vi "Calculate Forces.vi"(7 "Integrator Reset":bool, 8 "error in (no error)":errorcluster, 10 "Vessel in":refnum<class "Vessel.lvclass">, 11 "Joystick Controller in":refnum<class "Joystick Controller.lvclass">) -> (0 "error out":errorcluster, 2 "Vessel out":refnum<class "Vessel.lvclass">, 3 "Joystick Controller out":refnum<class "Joystick Controller.lvclass">)   [LabVIEW 2014, in "Controller Library.lvlib" / "Joystick Controller.lvclass"]
doc: "This VI calculates the forces in each controlled degree of freedom direction to follow a desired path or point."
uses:
  Joystick Controller.lvclass
  ROV/Vessel.lvclass
  <vilib>/addons/control/pid/pid.llb/PID (DBL).vi
  Supervisor/Supervisor.lvclass
  <vilib>/addons/control/pid/NI_PID_pid.lvlib
panel:
  in  "PID gains depth":T1={"proportional gain (Kc)"=500.0, "integral time (Ti, min)"=0.83, "derivative time (Td, min)"=0.01} {"derivative time (Td, min)" format="%.3f"; "integral time (Ti, min)" format="%.3f"; "proportional gain (Kc)" format="%.3f"}
  in  "PID gains head":T1={"proportional gain (Kc)"=150.0, "integral time (Ti, min)"=0.5, "derivative time (Td, min)"=0.008} {"derivative time (Td, min)" format="%.3f"; "integral time (Ti, min)" format="%.3f"; "proportional gain (Kc)" format="%.3f"}
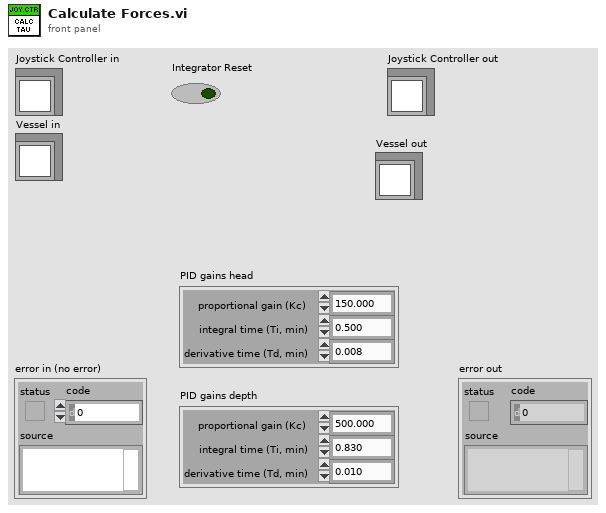
[diagram p1: front panel]
types:
  T1 = cluster{"proportional gain (Kc)":dbl, "integral time (Ti, min)":dbl, "derivative time (Td, min)":dbl}
  T2 = cluster{"Button 1":bool, "Button 2":bool, "Button 3":bool, "Button 4":bool, "Button 5":bool, "Button 6":bool, "Button 7":bool, "Button 8":bool, "Button 9":bool, "Button 10":bool, "Button 11":bool, "Button 12":bool, "POV Direction":i32}
  T3 = cluster{"Measured":cluster{"Eta":dbl[], "Nu":dbl[], "Eta Dot":dbl[], "Nu Dot":dbl[]}, "Estimated":cluster{"Eta":dbl[], "Nu":dbl[], "Eta Dot":dbl[], "Nu Dot":dbl[]}, "Desired":cluster{"Eta":dbl[], "Nu":dbl[], "Eta Dot":dbl[], "Nu Dot":dbl[]}, "Previous Desired":cluster{"Eta":dbl[], "Nu":dbl[], "Eta Dot":dbl[], "Nu Dot":dbl[]}, "tau":dbl[], "Altitude":cluster{"Measured":dbl, "Estimated":dbl, "Desired":dbl, "Previous Desired":dbl, "Approximated":dbl, "grad F":dbl[]}, "rpm":dbl[], "Attitude":cluster{"Theta Measured":dbl[], "Theta Estimated":dbl[], "Omega Measured":dbl[], "Omega Estimated":dbl[], "Gyro Bias":dbl[]}}
  T4 = cluster{"Axis Translation":cluster{"X-Axis":dbl, "Y-Axis":dbl, "Z-Axis":dbl}, "Axis Rotation":cluster{"X-Axis":dbl, "Y-Axis":dbl, "Z-Axis":dbl}}
  T5 = cluster{"Light 1":bool, "Light 2":bool, "Light 3":bool, "Light 4":bool, "HMI 1":bool, "HMI 2":bool, "Light Intensity 1":i32, "Light Intensity 2":i32, "Light Intensity 3":i8}
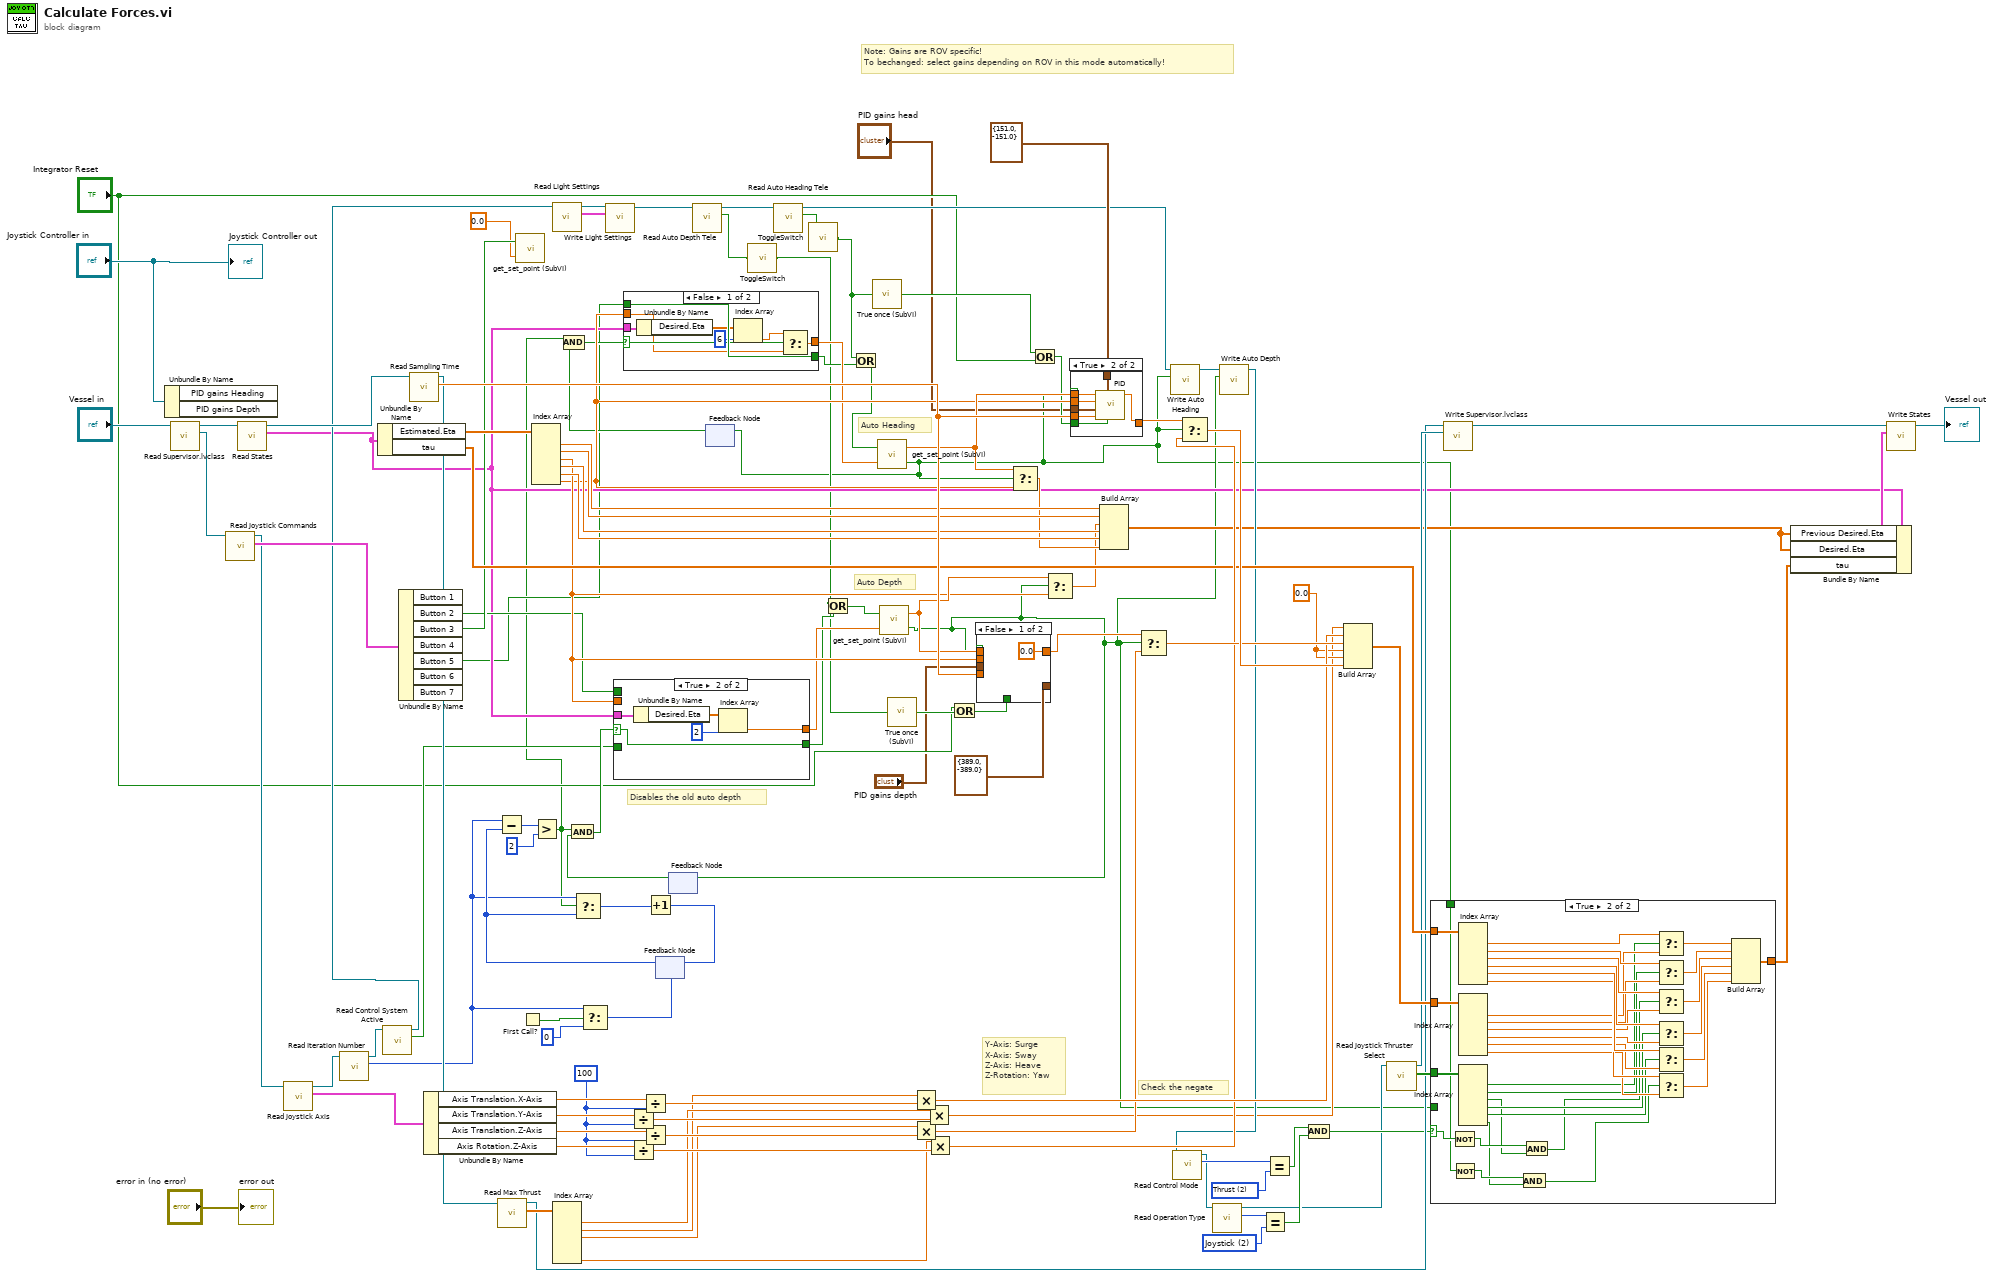
[diagram p0: block diagram]
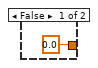
[diagram p2: hidden frame]
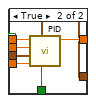
[diagram p3: hidden frame]
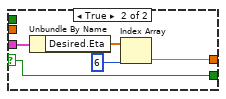
[diagram p4: hidden frame]
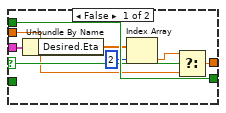
[diagram p5: hidden frame]
diagram:
  w66 = u16 2 items=["Tracking", "DP", "Joystick"] ("Operation Type")
  w68 = u16 2 items=["Position", "Velocity", "Thrust"] ("Control Mode")
  w85 = 0.0
  w97 = 100
  # "Note: Gains are ROV specific! \nTo bechanged: select gains depending on ROV in this mode automatically!"
  # "Disables the old auto depth"
  # "Check the negate"
  # "Y-Axis: Surge\nX-Axis: Sway\nZ-Axis: Heave\nZ-Rotation: Yaw"
  # "Auto Depth"
  # "Auto Heading"
  n1 = Unbundle By Name("Joystick Controller in") -> ()  [unwired: 2 out]
  n2 = call "Read Supervisor.lvclass.vi"("Vessel in"="Vessel in") -> ("Supervisor.lvclass"=w78:refnum<class "Supervisor.lvclass">, "Vessel out"=w113:refnum<class "Vessel.lvclass">)  [unwired: 8 in, 1 out]
  n3 = call-dynamic "Read Joystick Commands.vi"("Supervisor in"=w78) -> ("Joystick Commands"=w112:T2, "Supervisor out"=w77:refnum<class "Supervisor.lvclass">)  [unwired: 8 in, 1 out]
  n4 = call-dynamic "Read States.vi"("Vessel in"=w113) -> ("States"=w27:T3, "Vessel out"=w109:refnum<class "Vessel.lvclass">)  [unwired: 8 in, 1 out]
  n5 = call-dynamic "Read Joystick Axis.vi"("Supervisor in"=w77) -> ("Joystick Axis"=w103:T4, "Supervisor out"=w44:refnum<class "Supervisor.lvclass">)  [unwired: 8 in, 1 out]
  n6 = call-dynamic "Read Iteration Number.vi"("Supervisor in"=w44) -> ("Iteration Number"=w39:i32, "Supervisor out"=w32:refnum<class "Supervisor.lvclass">)  [unwired: 8 in, 1 out]
  n7 = Unbundle By Name(w27) -> ("Estimated.Eta"=w111:dbl[], "tau"=w84:dbl[])
  n8 = call-dynamic "Read Control System Active.vi"("Supervisor in"=w32) -> ("Control System Active"=w30:bool, "Supervisor out"=w31:refnum<class "Supervisor.lvclass">)  [unwired: 8 in, 1 out]
  n9 = Unbundle By Name(w112) -> ("Button 2"=w33:bool, "Button 3"=w80:bool, "Button 5"=w3:bool)  [unwired: 4 out]
  n10 = call-dynamic "Read Sampling Time.vi"("Vessel in"=w109) -> ("Sampling Time"=w108:dbl, "Vessel out"=w74:refnum<class "Vessel.lvclass">)  [unwired: 8 in, 1 out]
  n11 = Unbundle By Name(w103) -> ("Axis Translation.X-Axis"=w101:dbl, "Axis Translation.Y-Axis"=w100:dbl, "Axis Translation.Z-Axis"=w99:dbl, "Axis Rotation.Z-Axis"=w98:dbl)
  n12 = call "Read Max Thrust.vi"("Vessel in"=w74) -> ("Max Thrust"=w102:dbl[], "Vessel out"=w72:refnum<class "Vessel.lvclass">)  [unwired: 8 in, 1 out]
  n13 = call "get_set_point (SubVI).vi"("set point in"=0.0, "auto set  in"=w80) -> ()  [unwired: 2 out]
  n14 = First Call?() -> (First Call?: T/F=w47:bool)
  n15 = Index Array(array=w111) -> (element #1=w56:dbl, element #2=w55:dbl, element #3=w35:dbl, element #4=w54:dbl, element #5=w53:dbl, element #6=w29:dbl)  [unwired: 6 in]
  n16 = call-dynamic "Read Light Settings.vi"("Supervisor in"=w31) -> ("Light Settings"=w24:T5, "Supervisor out"=w76:refnum<class "Supervisor.lvclass">)  [unwired: 8 in, 1 out]
  n17 = Index Array(array=w102) -> (element #1=w92:dbl, element #2=w91:dbl, element #3=w90:dbl, element #6=w89:dbl)  [unwired: 6 in, 2 out]
  n18 = Select(t=w39, s=w47, f=0) -> (s? t:f=w45:i32)
  n19 = call-dynamic "Write Light Settings.vi"("Light Settings"=w24, "Supervisor in"=w76) -> ("Supervisor out"=w22:refnum<class "Supervisor.lvclass">)  [unwired: 8 in, 1 out]
  n20 = Divide(x=w100, y=w97) -> (x/y=w95:dbl)
  n21 = Divide(x=w98, y=w97) -> (x/y=w93:dbl)
  n22 = Divide(x=w101, y=w97) -> (x/y=w96:dbl)
  n23 = Divide(x=w99, y=w97) -> (x/y=w94:dbl)
  n24 = feedback #1(w45) -> (w40:i32)
  n25 = Subtract(x=w39, y=w40) -> (x-y=w43:i32)
  n26 = Greater?(x=w43, y=2) -> (0:w1:bool)
  n27 = Select(t=w39, s=w1, f=w40) -> (s? t:f=w38:i32)
  n28 = Increment(x=w38) -> (x+1=w37:i32)
  n29 = feedback-in #1(w37) -> ()
  n30 = feedback #2() -> (w41:bool)  [unwired: 1 in]
  n31 = And(x=w1, y=w41) -> (x .and. y?=w36:bool)
  n32 = case shown="True" w36 {
    selector: w36 -> [w122 w124]
    tunnel: w27 -> [w119 w128]
    tunnel: [w120 w125] -> w34
    tunnel: w35 -> [w121 _]
    tunnel: w33 -> [w123 _]
    tunnel: [w123 w124] -> w19
    tunnel: w30 -> [_ _]
    frame False {
      n33 = Unbundle By Name(w119) -> ("Desired.Eta"=w118:dbl[])
      n34 = Index Array(array=w118, index=2) -> (element=w116:dbl)
      n35 = Select(t=w116, s=w122, f=w121) -> (s? t:f=w120:dbl)
    }
    frame True {
      n36 = Unbundle By Name(w128) -> ("Desired.Eta"=w127:dbl[])
      n37 = Index Array(array=w127, index=2) -> (element=w125:dbl)
    }
  }
  n38 = call-dynamic "Read Auto Depth Tele.vi"("Supervisor in"=w22) -> ("Auto Depth Tele"=w15:bool, "Supervisor out"=w21:refnum<class "Supervisor.lvclass">)  [unwired: 8 in, 1 out]
  n39 = feedback #3() -> (w26:bool)  [unwired: 1 in]
  n40 = And(x=w1, y=w26) -> (x .and. y?=w25:bool)
  n41 = case shown="False" w25 {
    selector: w25 -> [w135 w137]
    tunnel: w27 -> [w132 w141]
    tunnel: [w133 w138] -> w28
    tunnel: w29 -> [w134 _]
    tunnel: w3 -> [w136 _]
    tunnel: [w136 w137] -> w17
    frame False {
      n42 = Unbundle By Name(w132) -> ("Desired.Eta"=w131:dbl[])
      n43 = Index Array(array=w131, index=6) -> (element=w129:dbl)
      n44 = Select(t=w129, s=w135, f=w134) -> (s? t:f=w133:dbl)
    }
    frame True {
      n45 = Unbundle By Name(w141) -> ("Desired.Eta"=w140:dbl[])
      n46 = Index Array(array=w140, index=6) -> (element=w138:dbl)
    }
  }
  n47 = call "ToggleSwitch.vi"("Input"=w15) -> ("Output"=w10:bool)
  n48 = call-dynamic "Read Auto Heading Tele.vi"("Supervisor in"=w21) -> ("Auto Heading Tele"=w14:bool, "Supervisor out"=w23:refnum<class "Supervisor.lvclass">)  [unwired: 8 in, 1 out]
  n49 = call "ToggleSwitch.vi"("Input"=w14) -> ("Output"=w13:bool)
  n50 = Or(x=w10, y=w19) -> (x .or. y?=w18:bool)
  n51 = Or(x=w13, y=w17) -> (x .or. y?=w16:bool)
  n52 = call "True once (SubVI).vi"("Automatic"=w13) -> ("Boolean"=w12:bool)
  n53 = call "get_set_point (SubVI).vi"("set point in"=w28, "auto set  in"=w16) -> ("auto set"=w2:bool, "set point"=w52:dbl)
  n54 = feedback-in #3(w2) -> ()
  n55 = call "get_set_point (SubVI).vi"("set point in"=w34, "auto set  in"=w18) -> ("auto set"=w4:bool, "set point"=w50:dbl)
  n56 = feedback-in #2(w4) -> ()
  n57 = call "True once (SubVI).vi"("Automatic"=w10) -> ("Boolean"=w9:bool)
  n58 = Multiply(x=w91, y=w96) -> (x*y=w88:dbl)
  n59 = Multiply(x=w90, y=w94) -> (x*y=w87:dbl)
  n60 = Multiply(x=w92, y=w95) -> (x*y=w20:dbl)
  n61 = Multiply(x=w89, y=w93) -> (x*y=w86:dbl)
  n62 = Or(x="Integrator Reset", y=w9) -> (x .or. y?=w7:bool)
  n63 = case shown="False" w4 {
    tunnel: w108 -> [_ w149]
    tunnel: [0.0 ("output") w148] -> w106
    tunnel: cluster{"output high":dbl, "output low":dbl} {"output high"=389.0, "output low"=-389.0} ("output range") -> [_ w147]
    tunnel: w50 -> [_ w146]
    tunnel: w35 -> [_ w145]
    tunnel: w7 -> [_ w144]
    tunnel: "PID gains depth" -> [_ w143]
    frame False {
    }
    frame True {
      n64 = call-poly <vilib>:"PID.vi"("reinitialize? (F)"=w144, "output range"=w147, "dt (s)"=w149, "PID gains"=w143, "process variable"=w145, "setpoint"=w146) -> ("output"=w148:dbl)  [unwired: 4 in, 1 out]
    }
  }
  n65 = Select(t=w52, s=w2, f=w29) -> (s? t:f=w51:dbl)
  n66 = Or(x=w12, y="Integrator Reset") -> (x .or. y?=w11:bool)
  n67 = Select(t=w50, s=w4, f=w35) -> (s? t:f=w49:dbl)
  n68 = case shown="True" w2 {
    tunnel: cluster{"output high":dbl, "output low":dbl} {"output high"=151.0, "output low"=-151.0} ("output range") -> [_ w157]
    tunnel: w108 -> [_ w156]
    tunnel: [0.0 ("output") w155] -> w107
    tunnel: w52 -> [_ w154]
    tunnel: w29 -> [_ w153]
    tunnel: w11 -> [_ w152]
    tunnel: "PID gains head" -> [_ w151]
    frame False {
    }
    frame True {
      n69 = call-poly <vilib>:"PID.vi"("reinitialize? (F)"=w152, "output range"=w157, "dt (s)"=w156, "PID gains"=w151, "process variable"=w153, "setpoint"=w154) -> ("output"=w155:dbl)  [unwired: 4 in, 1 out]
    }
  }
  n70 = Build Array(w56, w55, w49, w54, w53, w51) -> (w48:dbl[])
  n71 = Select(t=w106, s=w4, f=w87) -> (s? t:f=w104:dbl)
  n72 = call-dynamic "Write Auto Heading.vi"("Auto Heading"=w2, "Supervisor in"=w23) -> ("Supervisor out"=w75:refnum<class "Supervisor.lvclass">)  [unwired: 8 in, 1 out]
  n73 = Select(t=w107, s=w2, f=w86) -> (s? t:f=w105:dbl)
  n74 = call-dynamic "Write Auto Depth.vi"("Auto Depth"=w4, "Supervisor in"=w75) -> ("Supervisor out"=w62:refnum<class "Supervisor.lvclass">)  [unwired: 8 in, 1 out]
  n75 = call-dynamic "Read Control Mode.vi"("Supervisor in"=w62) -> ("Control Mode"=w69:u16, "Supervisor out"=w61:refnum<class "Supervisor.lvclass">)  [unwired: 8 in, 1 out]
  n76 = call-dynamic "Read Operation Type.vi"("Supervisor in"=w61) -> ("Operation Type"=w67:u16, "Supervisor out"=w60:refnum<class "Supervisor.lvclass">)  [unwired: 8 in, 1 out]
  n77 = Equal?(x=w67, y=w66) -> (x = y?=w64:bool)
  n78 = Equal?(x=w69, y=w68) -> (x = y?=w65:bool)
  n79 = And(x=w65, y=w64) -> (x .and. y?=w63:bool)
  n80 = Build Array(w20, w88, w104, w85, w85, w105) -> (w83:dbl[])
  n81 = call-dynamic "Read Joystick Thruster Select.vi"("Supervisor in"=w60) -> ("Joystick Thruster Select"=w82:bool[], "Supervisor out"=w73:refnum<class "Supervisor.lvclass">)  [unwired: 8 in, 1 out]
  n82 = case shown="True" w63 {
    selector: w63 -> [_ w166]
    tunnel: w84 -> [_ w192]
    tunnel: w83 -> [w158 w191]
    tunnel: w82 -> [_ w178]
    tunnel: [w158 w167] -> w81
    tunnel: w4 -> [_ _]
    tunnel: w2 -> [_ w162]
    frame False {
    }
    frame True {
      n83 = Not(x=w166) -> (.not. x?=w165:bool)
      n84 = Not(x=w162) -> (.not. x?=w161:bool)
      n85 = Index Array(array=w192) -> (element #1=w190:dbl, element #2=w189:dbl, element #3=w188:dbl, element #4=w187:dbl, element #5=w186:dbl, element #6=w185:dbl)  [unwired: 6 in]
      n86 = Index Array(array=w191) -> (element #1=w184:dbl, element #2=w183:dbl, element #3=w182:dbl, element #4=w181:dbl, element #5=w180:dbl, element #6=w179:dbl)  [unwired: 6 in]
      n87 = Index Array(array=w178) -> (element #1=w177:bool, element #2=w176:bool, element #3=w164:bool, element #4=w175:bool, element #5=w174:bool, element #6=w160:bool)  [unwired: 6 in]
      n88 = And(x=w161, y=w160) -> (x .and. y?=w159:bool)
      n89 = And(x=w165, y=w164) -> (x .and. y?=w163:bool)
      n90 = Select(t=w190, s=w177, f=w184) -> (s? t:f=w173:dbl)
      n91 = Select(t=w189, s=w176, f=w183) -> (s? t:f=w172:dbl)
      n92 = Select(t=w188, s=w163, f=w182) -> (s? t:f=w171:dbl)
      n93 = Select(t=w187, s=w175, f=w181) -> (s? t:f=w170:dbl)
      n94 = Select(t=w186, s=w174, f=w180) -> (s? t:f=w169:dbl)
      n95 = Select(t=w185, s=w159, f=w179) -> (s? t:f=w168:dbl)
      n96 = Build Array(w173, w172, w171, w170, w169, w168) -> (w167:dbl[])
    }
  }
  n97 = call "Write Supervisor.lvclass.vi"("Supervisor.lvclass"=w73, "Vessel in"=w72) -> ("Vessel out"=w71:refnum<class "Vessel.lvclass">)  [unwired: 8 in, 1 out]
  n98 = Bundle By Name(cluster=w27, "Previous Desired.Eta"=w48, "Desired.Eta"=w48, "tau"=w81) -> (w70:T3)
  n99 = call-dynamic "Write States.vi"("States"=w70, "Vessel in"=w71) -> ("Vessel out"=→"Vessel out":refnum<class "Vessel.lvclass">)  [unwired: 8 in, 1 out]
  "error out" <- "error in (no error)"
  "Joystick Controller out" <- "Joystick Controller in"
